vi "Average.vi"(10 "y":dbl, 11 "x":dbl) -> (3 "x/y":dbl)   [LabVIEW 2013]
doc: "Takes average of 2 numbers"
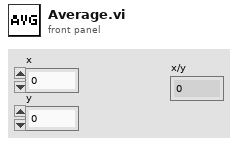
[diagram p1: front panel]
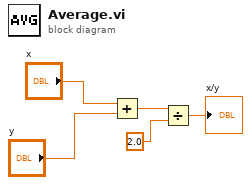
[diagram p0: block diagram]
diagram:
  n1 = Add(x="x", y="y") -> (x+y=w2:dbl)
  n2 = Divide(x=w2, y=2.0) -> (x/y=→"x/y":dbl)
